vi "E09_FeedbackNode EMMA.vi"() -> ()   [LabVIEW 2026]
panel:
  in  "stop":bool
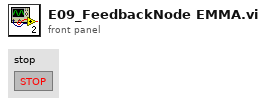
[diagram p1: front panel]
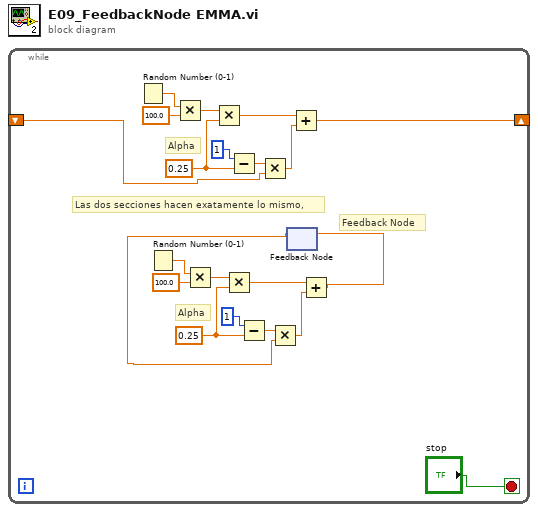
[diagram p0: block diagram]
diagram:
  n1 = while {
    shift-right: [w14] -> _
    shift-left: _ -> [w11]
    stop <- "stop" stop-if-true
    w6 = 0.25
    w16 = 0.25
    # "Feedback Node"
    # "Las dos secciones hacen exatamente lo mismo,"
    # "Alpha"
    # "Alpha"
    n2 = Random Number (0-1)() -> (number: 0 to 1=w19:dbl)
    n3 = Random Number (0-1)() -> (number: 0 to 1=w9:dbl)
    n4 = Multiply(x=w19, y=100.0) -> (x*y=w18:dbl)
    n5 = Multiply(x=w9, y=100.0) -> (x*y=w8:dbl)
    n6 = Multiply(x=w18, y=w16) -> (x*y=w15:dbl)
    n7 = Multiply(x=w8, y=w6) -> (x*y=w5:dbl)
    n8 = Subtract(x=1, y=w16) -> (x-y=w13:dbl)
    n9 = Subtract(x=1, y=w6) -> (x-y=w4:dbl)
    n10 = Multiply(x=w13, y=w11) -> (x*y=w12:dbl)
    n11 = feedback #1() -> (w1:dbl)  [unwired: 1 in]
    n12 = Multiply(x=w4, y=w1) -> (x*y=w3:dbl)
    n13 = Add(x=w15, y=w12) -> (x+y=w14:dbl)
    n14 = Add(x=w5, y=w3) -> (x+y=w2:dbl)
    n15 = feedback-in #1(w2) -> ()
  }
